vi "AndorSaveasSif_Ver2.vi"(5 "Phase":i32, 6 "Time":string, 7 "Dir":i32, 8 "error in":errorcluster, 9 "No.":i32, 10 "KinNumber":i32=10, 11 "FilePath":string="C:\\Users\\light\\Desktop\\Andor\\data") -> (0 "error out":errorcluster, 3 "SaveStatus":bool)   [LabVIEW 2014]
uses:
  <userlib>/atmcd64d.llb/Spool_method typedef.ctl
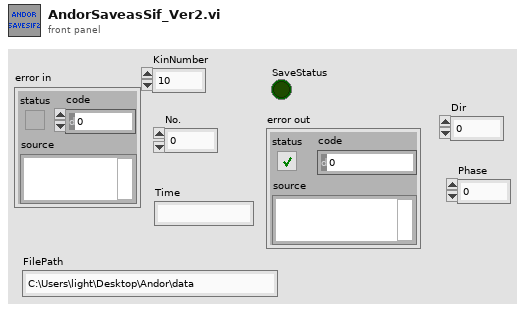
[diagram p1: front panel]
types:
  T1 = typedef "Spool_method typedef.ctl" = enum16{"32-bit", "Depends", "16-bit", "Multiple Directory", "Spool to RAM disk", "16-bit FITS", "SIF", "16-buit TIFF", "Multiple Directory Compressed"}
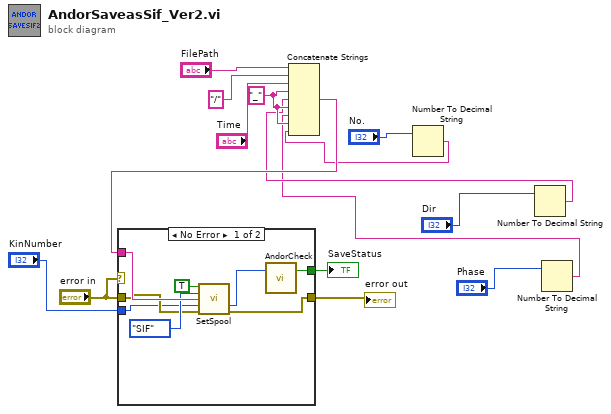
[diagram p0: block diagram]
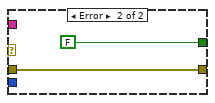
[diagram p2: hidden frame]
diagram:
  w4 = "_" ("string")
  n1 = Number To Decimal String(number="No.") -> (decimal integer string=w1:string)  [unwired: 1 in]
  n2 = Number To Decimal String(number="Dir") -> (decimal integer string=w3:string)  [unwired: 1 in]
  n3 = Number To Decimal String(number="Phase") -> (decimal integer string=w2:string)  [unwired: 1 in]
  n4 = Concatenate Strings("FilePath", "/" ("string"), "Time", w4, w3, w4, w2, w4, w1) -> (w10:string)
  n5 = case shown="No Error" "error in" {
    tunnel: "error in" -> [w19 w24]
    tunnel: [w23 FALSE ("Status")] -> w14
    tunnel: [w17 w24] -> w13
    tunnel: w10 -> [w22 _]
    tunnel: "KinNumber" -> [w18 _]
    frame No Error {
      n6 = call <userlib>:"SetSpool.vi"("active"=TRUE, "method"=Spool_method_typedef."SIF", "name"=w22, "framebuffersize (10)"=w18, "error in (no error)"=w19) -> ("DLL error code"=w16:u32, "error out"=w17:errorcluster)  [unwired: 9 in]
      n7 = call "AndorCheck.vi"("Input"=w16) -> ("Status"=w23:bool)  [unwired: 1 in, 1 out]
    }
    frame Error {
    }
  }
  "SaveStatus" <- w14
  "error out" <- w13
